vi "A-Weight Spectrum - DEV ONLY.vi"(0 "Max Frequency (Hz)":dbl=20000.0, 2 "Frequency Resolution (Hz)":dbl=1.0) -> ()   [LabVIEW 2020, in "GSwFormDSP.lvclass"]
uses:
  GSwFormDSP.lvclass
panel:
  out "XY Graph 2":cluster{dbl[], dbl[]}(graph)
  out "XY Graph":cluster{dbl[], dbl[]}(graph)
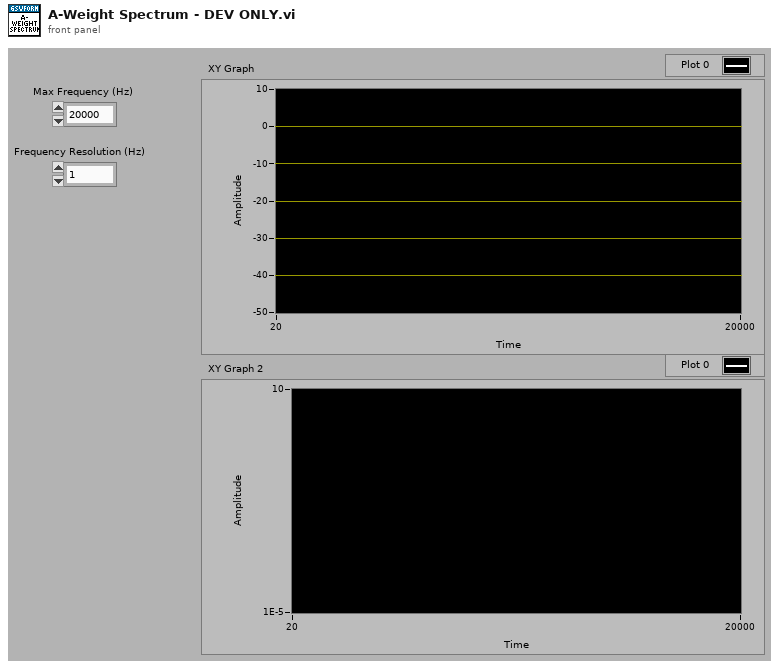
[diagram p1: front panel]
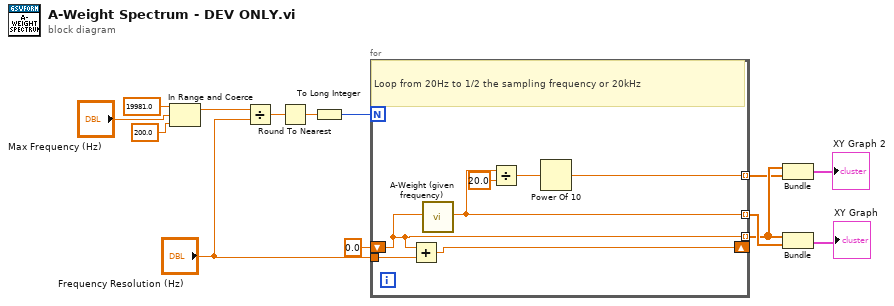
[diagram p0: block diagram]
diagram:
  n1 = In Range and Coerce(upper limit=19981.0, x="Max Frequency (Hz)", lower limit=200.0) -> (coerced(x)=w12:dbl)  [unwired: 1 out]
  n2 = Divide(x=w12, y="Frequency Resolution (Hz)") -> (x/y=w11:dbl)
  n3 = Round To Nearest(number=w11) -> (nearest integer value=w10:dbl)
  n4 = To Long Integer(number=w10) -> (32bit integer=w9:i32)
  n5 = for {
    N: w9 -> [_]
    shift-right: [w20] -> _
    shift-left: 0.0 ("lower limit") -> [w19]
    tunnel: "Frequency Resolution (Hz)" -> [w21]
    tunnel: [w19] -> w3 mode=indexing
    tunnel: [w18] -> w6 mode=indexing
    tunnel: [w15] -> w2 mode=indexing
    # "Loop from 20Hz to 1/2 the sampling frequency or 20kHz"
    n6 = Add(x=w19, y=w21) -> (x+y=w20:dbl)
    n7 = call "A-Weight (given frequency).vi"("Frequency (Hz)"=w19) -> ("A-Weight (dB)"=w18:dbl)  [unwired: 18 in]
    n8 = Divide(x=w18, y=20.0) -> (x/y=w16:dbl)
    n9 = Power Of 10(x=w16) -> (10^x=w15:dbl)
  }
  n10 = Bundle(w3, w2) -> (→"XY Graph 2":cluster{dbl[], dbl[]})  [unwired: 1 in]
  n11 = Bundle(w3, w6) -> (→"XY Graph":cluster{dbl[], dbl[]})  [unwired: 1 in]
